vi "Serialize - JSON.vi"(8 "error in":errorcluster, 11 "PAS Cell Data in":refnum<class "PAS Cell Data.lvclass">) -> (0 "error out":errorcluster, 2 "Serialized JSON":string, 3 "PAS Cell Data out":refnum<class "PAS Cell Data.lvclass">)   [LabVIEW 2014, in "PAS Library.lvlib" / "PAS Cell Data.lvclass"]
uses:
  PAS Cell Data.lvclass
  <vilib>/Analysis/Matrix/Datatypes/RealMatrix.ctl
  PAS Cell Data.lvclass/PAS Cell Data.ctl
  <vilib>/Analysis/Matrix/NI_Matrix.lvlib
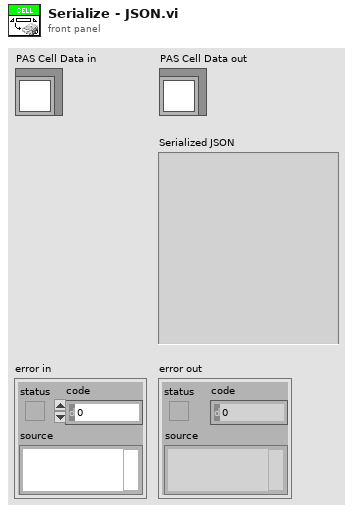
[diagram p1: front panel]
types:
  T1 = typedef "NI_Matrix.lvlib/RealMatrix.ctl" = dbl[][]
  T2 = cluster{"derived":cluster{"f0":sgl, "IA":sgl, "Q":sgl, "max":dbl[], "noiseLim":dbl, "ext":dbl}, "fitData":cluster{"parameters":dbl[], "covariance":T1}, "IABack":dbl, "FittedData":cluster{"Y":sgl[], "dt":dbl}, "MicFreq":cluster{"Y":sgl[], "dt":dbl}, "MicTime":cluster{"Y":i16[], "dt":dbl}, "PhotoDiode":cluster{"Y":i16[], "dt":dbl}, "lRMS":dbl}
  T3 = cluster{"f0":sgl, "IA":sgl, "Q":sgl, "max":dbl[], "noiseLim":dbl, "abs":dbl}
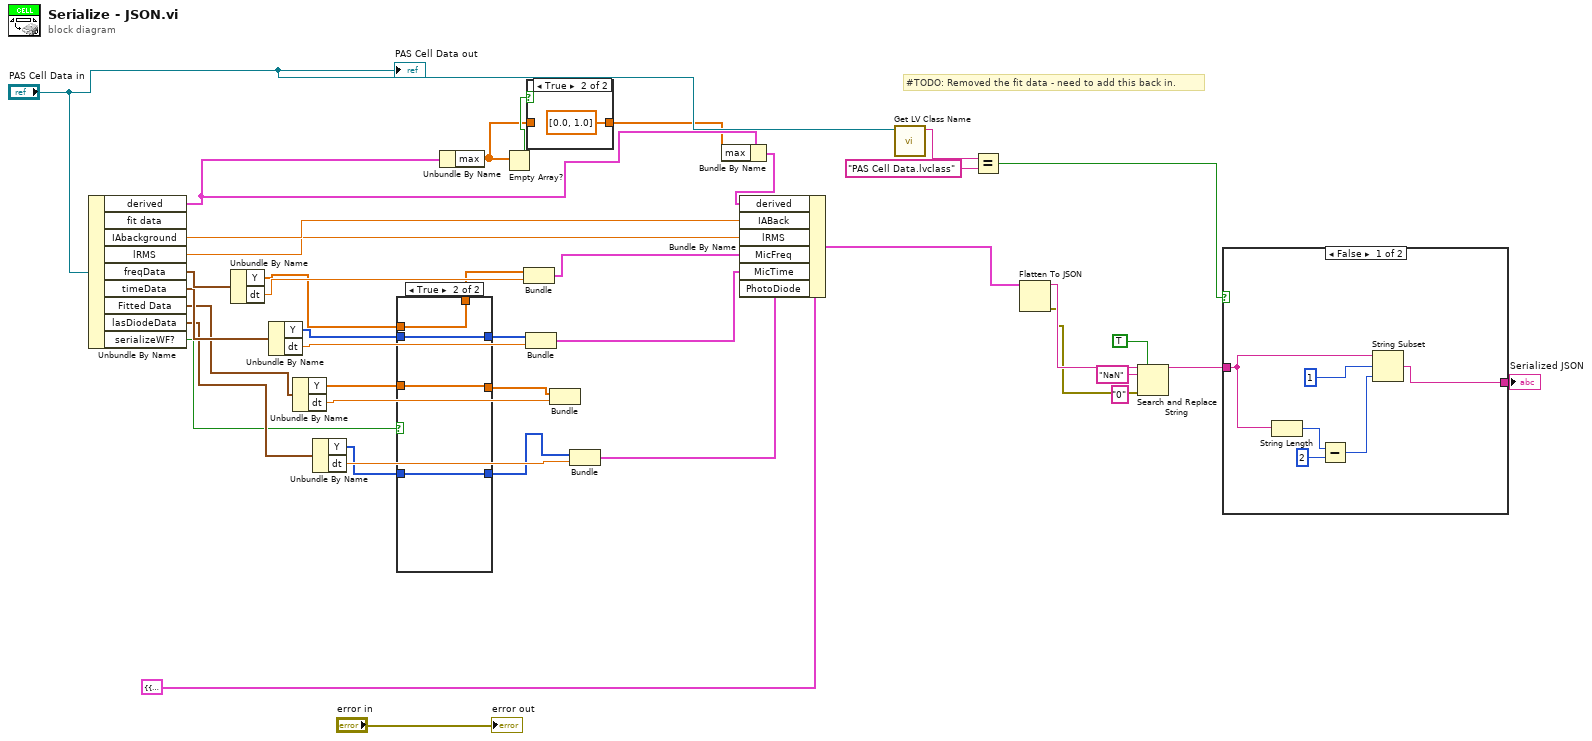
[diagram p0: block diagram]
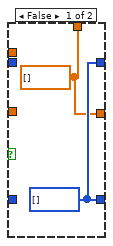
[diagram p2: hidden frame]
diagram:
  # "#TODO: Removed the fit data - need to add this back in."
  n1 = Unbundle By Name("PAS Cell Data in") -> ("derived"=w14:T3, "IAbackground"=w40:dbl, "lRMS"=w39:dbl, "freqData"=w38:waveform(sgl), "timeData"=w34:waveform(i16), "Fitted Data"=w31:waveform(sgl), "lasDiodeData"=w29:waveform(i16), "serializeWF?"=w9:bool)  [unwired: 1 out]
  n2 = Unbundle By Name(w38) -> ("Y"=w4:sgl[], "dt"=w37:dbl)
  n3 = Unbundle By Name(w34) -> ("Y"=w3:i16[], "dt"=w35:dbl)
  n4 = Unbundle By Name(w31) -> ("Y"=w2:sgl[], "dt"=w32:dbl)
  n5 = Unbundle By Name(w29) -> ("Y"=w1:i16[], "dt"=w30:dbl)
  n6 = case shown="True" w9 {
    tunnel: [w43 w44] -> w8
    tunnel: [w43 w46] -> w7
    tunnel: [w42 w47] -> w6
    tunnel: [w42 w45] -> w5
    tunnel: w4 -> [_ w47]
    tunnel: w3 -> [_ w46]
    tunnel: w2 -> [_ w45]
    tunnel: w1 -> [_ w44]
    frame False {
      w43 = i16[] [] ("Y")
      w42 = sgl[] [] ("Y")
    }
    frame True {
    }
  }
  n7 = Unbundle By Name(w14) -> ("max"=w15:dbl[])
  n8 = Empty Array?(array=w15) -> (empty?=w16:bool)
  n9 = Bundle("Y"=w6, "dt"=w37) -> (w36:cluster{"Y":sgl[], "dt":dbl})  [unwired: 1 in]
  n10 = Bundle("Y"=w7, "dt"=w35) -> (w33:cluster{"Y":i16[], "dt":dbl})  [unwired: 1 in]
  n11 = case shown="True" w16 {
    tunnel: w15 -> [w48 _]
    tunnel: [w48 dbl[] [0.0, 1.0] ("max")] -> w13
    frame False {
    }
    frame True {
    }
  }
  n12 = Bundle("Y"=w5, "dt"=w32) -> ()  [unwired: 1 in, 1 out]
  n13 = Bundle("Y"=w8, "dt"=w30) -> (w28:cluster{"Y":i16[], "dt":dbl})  [unwired: 1 in]
  n14 = Bundle By Name(cluster=w14, "max"=w13) -> (w12:T3)
  n15 = Bundle By Name(cluster=T2 {"derived"={"f0"=0.0, "IA"=0.0, "Q"=0.0, "max"=[0.0], "noiseLim"=0.0, "ext"=0.0}, "fitData"={"parameters"=[0.0], "covariance"=[[0.0, 0.0], [0.0, 0.0]]}, "IABack"=0.0, "FittedData"={"Y"=[0.0], "dt"=0.0}, "MicFreq"={"Y"=[0.0], "dt"=0.0}, "MicTime"={"Y"=[0], "dt"=0.0}, "PhotoDiode"={"Y"=[0], "dt"=0.0}, "lRMS"=0.0}, "derived"=w12, "IABack"=w40, "lRMS"=w39, "MicFreq"=w36, "MicTime"=w33, "PhotoDiode"=w28) -> (w27:T2)
  n16 = call <vilib>:"Get LV Class Name.vi"("object"="PAS Cell Data in") -> ("class name"=w22:string)  [unwired: 9 in, 1 out]
  n17 = Equal?(x=w22, y="PAS Cell Data.lvclass") -> (x = y?=w20:bool)
  n18 = Flatten To JSON(anything=w27) -> (JSON string=w26:string, 11:w11:errorcluster)  [unwired: 2 in]
  n19 = Search and Replace String(replace all?=TRUE ("replace all? (F)"), input string=w26, search string="NaN", replace string="0" ("replace string (\"\")"), error in=w11) -> (result string=w19:string)  [unwired: 3 in, 3 out]
  n20 = case shown="False" w20 {
    tunnel: w19 -> [w54 w56]
    tunnel: [w50 w56] -> w18
    frame False {
      n21 = String Length(string=w54) -> (length=w53:i32)
      n22 = Subtract(x=w53, y=2) -> (x-y=w51:i32)
      n23 = String Subset(string=w54, offset (0)=1, length (rest)=w51) -> (substring=w50:string)
    }
    frame True {
    }
  }
  "Serialized JSON" <- w18
  "error out" <- "error in"
  "PAS Cell Data out" <- "PAS Cell Data in"
